vi "put_tablecloths.vi"(8 "error in (no error)":errorcluster, 11 "tables in":refnum<class "ITable.lvclass">[](array[class])) -> (0 "error out":errorcluster, 2 "tablecloth results":string[](array[string]), 3 "tables out":refnum<class "ITable.lvclass">[](array[class]))   [LabVIEW 2021]
uses:
  ITable/ITable.lvclass
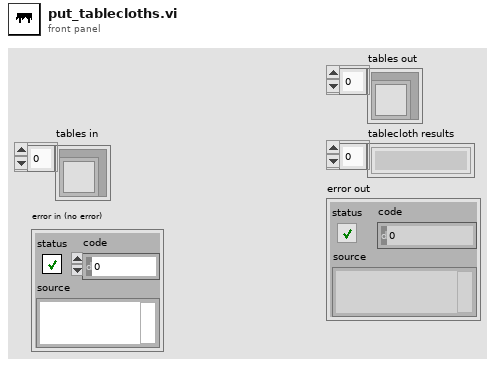
[diagram p1: front panel]
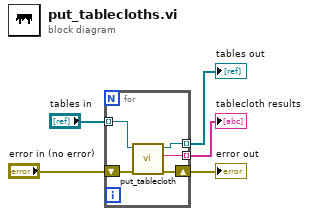
[diagram p0: block diagram]
diagram:
  n1 = for {
    tunnel: "tables in" -> [w10] mode=indexing
    shift-right: [w8] -> w1
    shift-left: "error in (no error)" -> [w9]
    tunnel: [w7] -> w2 mode=indexing
    tunnel: [w6] -> w3 mode=indexing
    n2 = call-dynamic "put_tablecloth.vi"("error in (no error)"=w9, "ITable in"=w10) -> ("error out"=w8:errorcluster, "result"=w7:string, "ITable out"=w6:refnum<class "ITable.lvclass">)  [unwired: 7 in]
  }
  "tables out" <- w3
  "tablecloth results" <- w2
  "error out" <- w1
